vi "TTA_MATLAB_RFIC_TX_Enable.vi"(0 "Channels":string[](array[combo]), 11 "error in":errorcluster) -> (4 "SuccessComm":bool[](array[boolean]), 15 "error out":errorcluster)   [LabVIEW 2016]
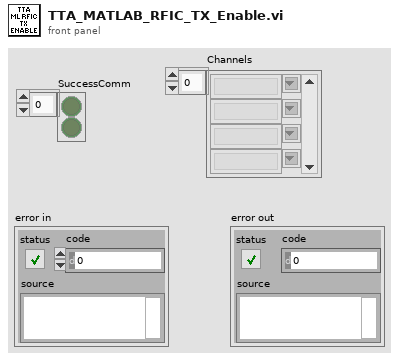
[diagram p1: front panel]
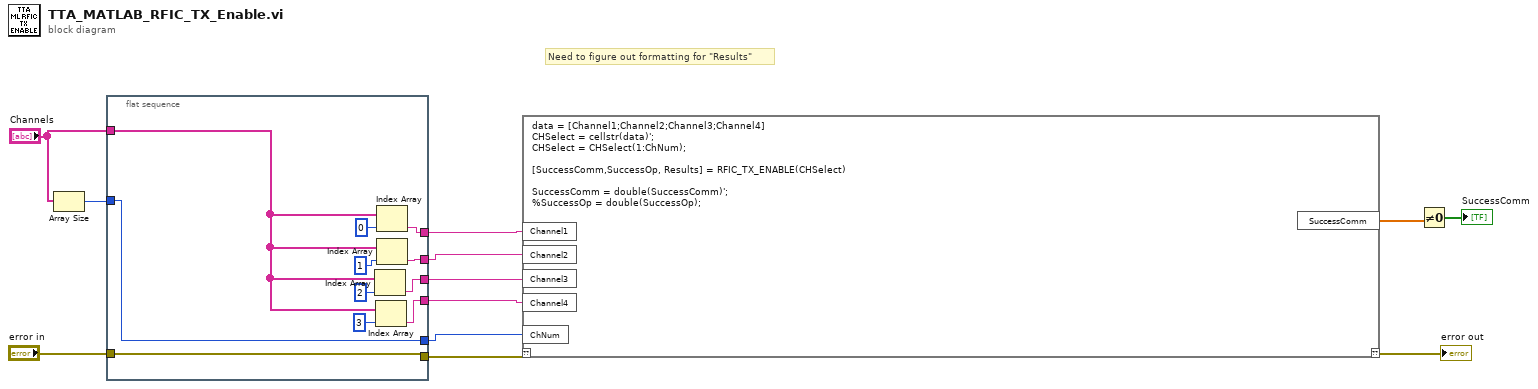
[diagram p0: block diagram]
diagram:
  # "Need to figure out formatting for \"Results\""
  n1 = Array Size(array="Channels") -> (size(s)=w8:i32)
  n2 = flat-sequence {
    tunnel: "error in" -> [w23]
    tunnel: [w22] -> w4
    tunnel: w8 -> [w16]
    tunnel: [w23] -> w6
    tunnel: "Channels" -> [w15]
    tunnel: [w19] -> w3
    tunnel: [w17] -> w2
    tunnel: [w16] -> w5
    tunnel: [w13] -> w1
    frame #0 {
      n3 = Index Array(array=w15, index=2) -> (element=w17:string)
      n4 = Index Array(array=w15, index=3) -> (element=w13:string)
      n5 = Index Array(array=w15, index=0) -> (element=w22:string)
      n6 = Index Array(array=w15, index=1) -> (element=w19:string)
    }
  }
  n7 = script code="data = [Channel1;Channel2;Channel3;Channel4]\nCHSelect = cellstr(data)';\nCHSelect = CHSelect(1:ChNum);\n\n[SuccessComm,SuccessOp, Results] = RFIC_TX_ENABLE(CHSelect)\n\nSuccessComm = double(SuccessComm)';\n%SuccessOp = double(SuccessOp);"("??"=w6, "Channel1"=w4, "ChNum"=w5, "Channel2"=w3, "Channel3"=w2, "Channel4"=w1) -> ("??"=→"error out":errorcluster, "SuccessComm"=w10:dbl[])
  n8 = Not Equal To 0?(x=w10) -> (x != 0?=→"SuccessComm":bool[])
